vi "Bed_control.vi"(11 "pulse steps":i32=6436 min=4 step=1) -> ()   [LabVIEW 2019]
uses:
  <vilib>/DAQmx/write.llb/DAQmx Write (Digital 1D Wfm NChan NSamp).vi
  <vilib>/DAQmx/read.llb/DAQmx Read (Digital Bool 1Line 1Point).vi
  <vilib>/DAQmx/create/channels.llb/DAQmx Create Channel (DO-Digital Output).vi
  <vilib>/DAQmx/create/channels.llb/DAQmx Create Channel (DI-Digital Input).vi
  <vilib>/DAQmx/configure/timing.llb/DAQmx Timing (Sample Clock).vi
  <vilib>/Waveform/DWDTOps.llb/DWDT Digital Size.vi
  <vilib>/Waveform/DWDTOps.llb/DWDT Uncompress Digital.vi
  <vilib>/DAQmx/miscellaneous.llb/DAQmx Fill In Error Info.vi
  global_variables.vi
panel:
  out "travel distance (mm)":dbl=643.6
  in  "Move bed 2":bool
  in  "latch switch line":tag="DAQ1/port0/line3"
  out "Homing in progress":bool
  out "duration of movement":dbl=38.616
  in  "output lines":tag="DAQ1/port0/line0:2"
  in  "pulse duration (T/2)":dbl=0.003 format="%#_13p"
  out "Position":dbl(slide)=6836.0 scale=0.0..8000.0
  in  "Maximum absolute position":i32=8000 format="%.0p"
  out "Absolute position (pulses)":i32=6836
  in  "Abort movement":bool
  in  "Go home!":bool
  in  "Move bed":bool
  out "pulses to move":i32=6436
  in  "stop":bool
  # "DAQ settings"
  # "Homing"
  # "Enables PDU automatically"
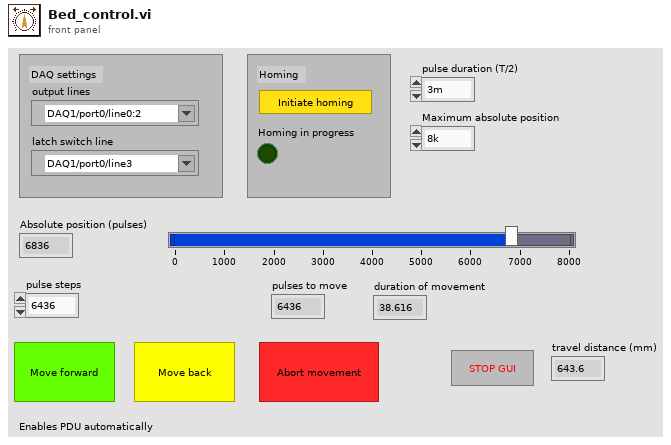
[diagram p1: front panel]
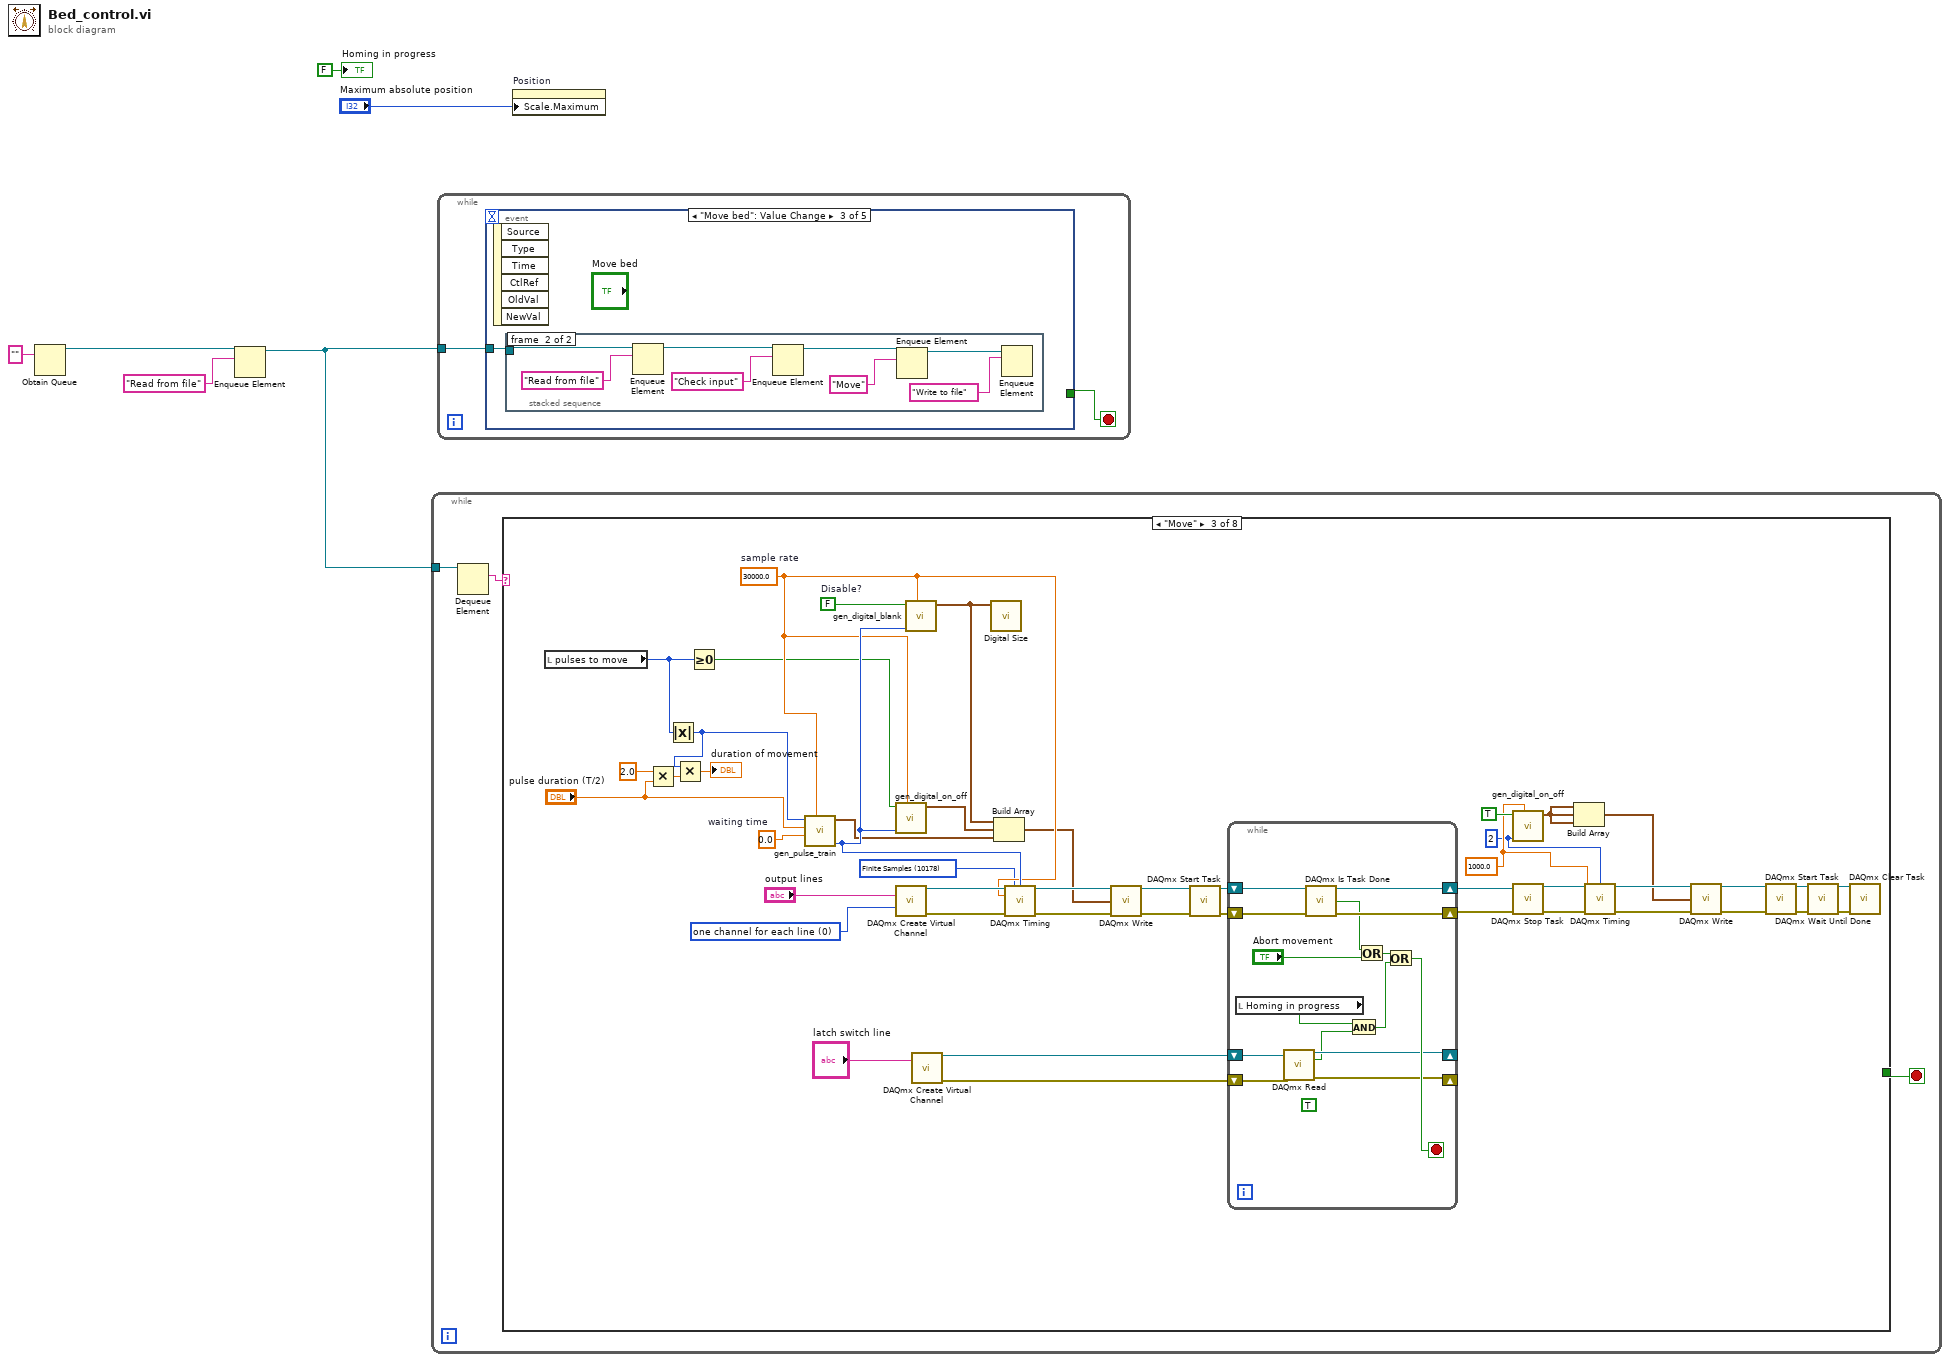
[diagram p0: block diagram]
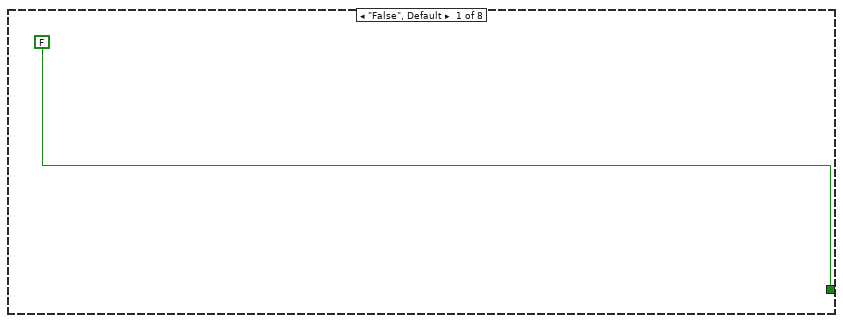
[diagram p2: hidden frame]
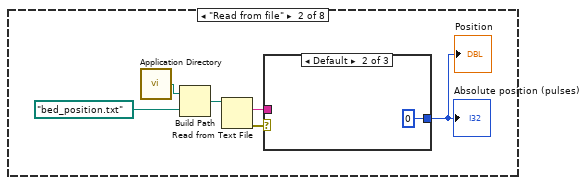
[diagram p3: hidden frame]
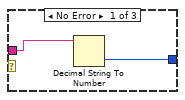
[diagram p4: hidden frame]
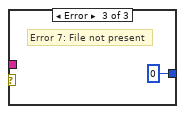
[diagram p5: hidden frame]
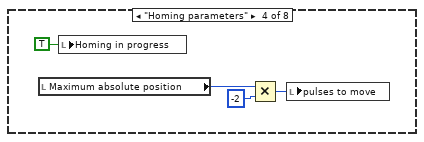
[diagram p6: hidden frame]
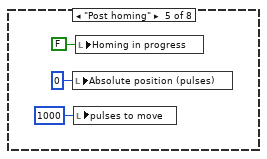
[diagram p7: hidden frame]
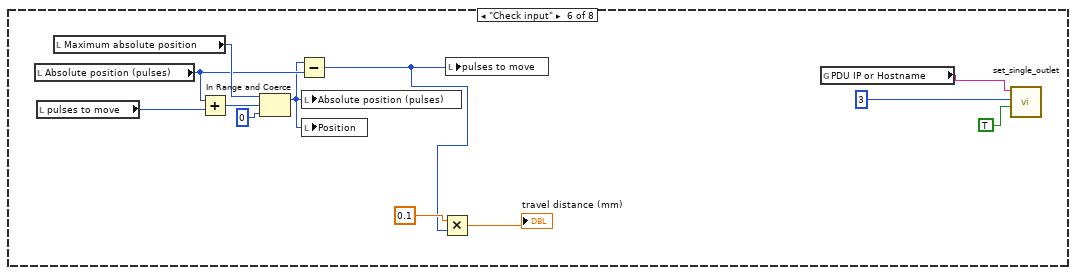
[diagram p8: hidden frame]
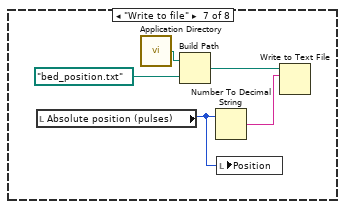
[diagram p9: hidden frame]
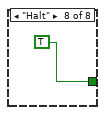
[diagram p10: hidden frame]
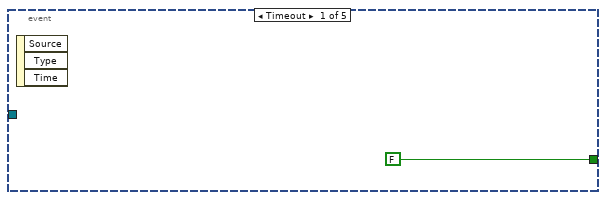
[diagram p11: hidden frame]
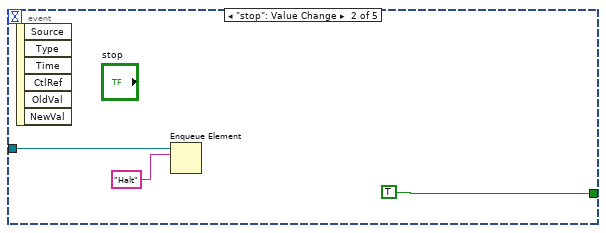
[diagram p12: hidden frame]
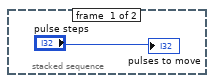
[diagram p13: hidden frame]
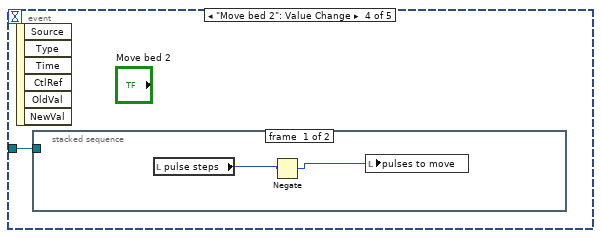
[diagram p14: hidden frame]
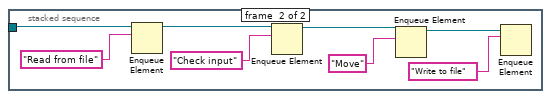
[diagram p15: hidden frame]
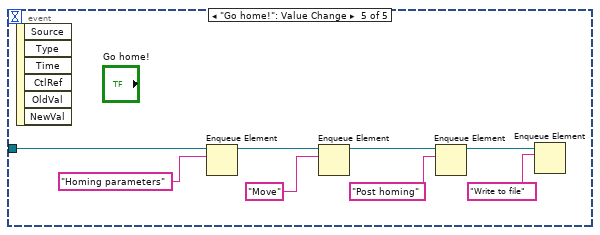
[diagram p16: hidden frame]
diagram:
  n1 = Obtain Queue(element data type="") -> (queue out=w5:refnum<queue>)  [unwired: 4 in, 2 out]
  n2 = Enqueue Element(queue=w5, element="Read from file") -> (queue out=w4:refnum<queue>)  [unwired: 2 in, 2 out]
  n3 = while {
    tunnel: w4 -> [w9]
    stop <- w7 stop-if-true
    n4 = Dequeue Element(queue=w9) -> (element=w8:string)  [unwired: 2 in, 3 out]
    n5 = case shown="\"Move\"" w8 {
      tunnel: [FALSE _ _ _ _ _ _ TRUE] -> w7
      frame "False", Default {
      }
      frame "Read from file" {
        n6 = call <vilib>:"Application Directory.vi"() -> ("Application Directory"=w13:path)
        n7 = Build Path(base path=w13, name or relative path=path "bed_position.txt" ("file (use dialog)")) -> (appended path=w14:path)
        n8 = Read from Text File(file (use dialog)=w14) -> (text=w16:string, error out=w15:errorcluster)  [unwired: 3 in, 2 out]
        n9 = case shown="Default" w15 {
          tunnel: w16 -> [w18 _ _]
          tunnel: [w17 0 0] -> w11
          frame No Error {
            n10 = Decimal String To Number(string=w18) -> (number=w17:i32)  [unwired: 2 in, 1 out]
          }
          frame Default {
          }
          frame Error {
            # "Error 7: File not present"
          }
        }
        "Absolute position (pulses)" <- w11
        "Position" <- w11
      }
      frame "Move" {
        w26 = 2 ("waveform length")
        w27 = 1000.0 ("rate")
        w51 = 0.0  # waiting time
        w56 = 30000.0  # sample rate
        w55 = FALSE  # Disable?
        w54 = 10178 items=["Finite Samples"=10178, "Continuous Samples"=10123, "Hardware Timed Single Point"=12522] ("sample mode")
        w52 = 0 items=["one channel for each line", "one channel for all lines"] ("line grouping")
        n11 = local read "pulses to move"() -> (w25:i32)
        n12 = Multiply(x=2.0, y="pulse duration (T/2)") -> (x*y=w47:dbl)
        n13 = Absolute Value(x=w25) -> (abs(x)=w48:i32)
        n14 = Multiply(x=w48, y=w47) -> (x*y=→"duration of movement":dbl)
        n15 = Greater Or Equal To 0?(x=w25) -> (x >= 0?=w50:bool)
        n16 = call "gen_pulse_train.vi"("sampling rate"=w56, "waiting time"=w51, "pulse width"="pulse duration (T/2)", "Number of pulses"=w48) -> ("waveform length"=w63:i32, "digital waveform out"=w61:digitalwaveform)  [unwired: 6 in]
        n17 = call "gen_digital_on_off.vi"("sampling rate"=w56, "waveform length"=w63, "On / Off"=w50) -> ("digital waveform"=w62:digitalwaveform)  [unwired: 8 in]
        n18 = call-poly <vilib>:"DAQmx Create Virtual Channel.vi"("lines"="output lines", "line grouping"=w52) -> ("task out"=w57:refnum<k21>, "error out"=w60:errorcluster)  [unwired: 12 in]
        n19 = call "gen_digital_blank.vi"("sampling rate"=w56, "waveform length"=w63, "On / Off"=w55) -> ("digital waveform"=w66:digitalwaveform)  [unwired: 8 in]
        n20 = call-poly <vilib>:"DAQmx Create Virtual Channel.vi"("lines"="latch switch line") -> ("task out"=w22:refnum<k21>, "error out"=w23:errorcluster)  [unwired: 13 in]
        n21 = call-poly <vilib>:"Digital Size.vi"("digital waveform in"=w66) -> ()  [unwired: 7 in, 4 out]
        n22 = Build Array(w66, w62, w61) -> (w21:digitalwaveform[])
        n23 = call-poly <vilib>:"DAQmx Timing.vi"("task/channels in"=w57, "sample mode"=w54, "samples per channel"=w63, "rate"=w56, "error in"=w60) -> ("task out"=w58:refnum<k21>, "error out"=w59:errorcluster)  [unwired: 9 in]
        n24 = call-poly <vilib>:"DAQmx Write.vi"("task/channels in"=w58, "data"=w21, "error in"=w59) -> ("task out"=w64:refnum<k21>, "error out"=w65:errorcluster)  [unwired: 10 in, 1 out]
        n25 = call <vilib>:"DAQmx Start Task.vi"("task/channels in"=w64, "error in"=w65) -> ("task out"=w44:refnum<k21>, "error out"=w43:errorcluster)  [unwired: 12 in]
        n26 = while {
          shift-right: [w78] -> w41
          shift-left: w43 -> [w80]
          shift-right: [w79] -> w42
          shift-left: w44 -> [w81]
          shift-right: [w70] -> _
          shift-left: w22 -> [w73]
          shift-right: [w71] -> _
          shift-left: w23 -> [w72]
          stop <- w74 stop-if-true
          (unwired) TRUE ("Abort movement")
          n27 = local read "Homing in progress"() -> (w69:bool)
          n28 = call-poly <vilib>:"DAQmx Read.vi"("task/channels in"=w73, "error in"=w72) -> ("task out"=w70:refnum<k21>, "data"=w67:bool, "error out"=w71:errorcluster)  [unwired: 11 in]
          n29 = call <vilib>:"DAQmx Is Task Done.vi"("task/channels in"=w81, "error in"=w80) -> ("task out"=w79:refnum<k21>, "task done?"=w76:bool, "error out"=w78:errorcluster)  [unwired: 11 in]
          n30 = And(x=w69, y=w67) -> (x .and. y?=w68:bool)
          n31 = Or(x=w76, y="Abort movement") -> (x .or. y?=w75:bool)
          n32 = Or(x=w75, y=w68) -> (x .or. y?=w74:bool)
        }
        n33 = call "gen_digital_on_off.vi"("sampling rate"=w27, "waveform length"=w26, "On / Off"=TRUE) -> ("digital waveform"=w30:digitalwaveform)  [unwired: 8 in]
        n34 = call <vilib>:"DAQmx Stop Task.vi"("task/channels in"=w42, "error in"=w41) -> ("task out"=w31:refnum<k21>, "error out"=w34:errorcluster)  [unwired: 12 in]
        n35 = Build Array(w30, w30, w30) -> (w29:digitalwaveform[])
        n36 = call-poly <vilib>:"DAQmx Timing.vi"("task/channels in"=w31, "samples per channel"=w26, "rate"=w27, "error in"=w34) -> ("task out"=w32:refnum<k21>, "error out"=w33:errorcluster)  [unwired: 10 in]
        n37 = call-poly <vilib>:"DAQmx Write.vi"("task/channels in"=w32, "data"=w29, "error in"=w33) -> ("task out"=w40:refnum<k21>, "error out"=w39:errorcluster)  [unwired: 10 in, 1 out]
        n38 = call <vilib>:"DAQmx Start Task.vi"("task/channels in"=w40, "error in"=w39) -> ("task out"=w38:refnum<k21>, "error out"=w37:errorcluster)  [unwired: 12 in]
        n39 = call <vilib>:"DAQmx Wait Until Done.vi"("task/channels in"=w38, "error in"=w37) -> ("task out"=w36:refnum<k21>, "error out"=w35:errorcluster)  [unwired: 12 in]
        n40 = call <vilib>:"DAQmx Clear Task.vi"("task in"=w36, "error in"=w35) -> ()  [unwired: 13 in, 1 out]
      }
      frame "Homing parameters" {
        n41 = local read "Maximum absolute position"() -> (w84:i32)
        n42 = local write "Homing in progress"(TRUE ("Homing in progress")) -> ()
        n43 = Multiply(x=w84, y=-2) -> (x*y=w82:i32)
        n44 = local write "pulses to move"(w82) -> ()
      }
      frame "Post homing" {
        n45 = local write "Absolute position (pulses)"(0 ("Absolute position (pulses)")) -> ()
        n46 = local write "pulses to move"(1000 ("pulses to move")) -> ()
        n47 = local write "Homing in progress"(FALSE ("Homing in progress")) -> ()
      }
      frame "Check input" {
        n48 = local read "Absolute position (pulses)"() -> (w98:i32)
        n49 = local read "pulses to move"() -> (w95:i32)
        n50 = local read "Maximum absolute position"() -> (w99:i32)
        n51 = Add(x=w98, y=w95) -> (x+y=w100:i32)
        n52 = In Range and Coerce(upper limit=w99, x=w100, lower limit=0) -> (coerced(x)=w97:i32)  [unwired: 1 out]
        n53 = Subtract(x=w97, y=w98) -> (x-y=w92:i32)
        n54 = local write "Absolute position (pulses)"(w97) -> ()
        n55 = local write "Position"(w97) -> ()
        n56 = Multiply(x=0.1, y=w92) -> (x*y=→"travel distance (mm)":dbl)
        n57 = local write "pulses to move"(w92) -> ()
        n58 = global read "global_variables.vi" "PDU IP or Hostname"() -> (w91:string)
        n59 = call "set_single_outlet.vi"("Switch state"=TRUE, "Outlet #"=3, "IP / Hostname"=w91) -> ()  [unwired: 9 in]
      }
      frame "Write to file" {
        n60 = local read "Absolute position (pulses)"() -> (w101:i32)
        n61 = call <vilib>:"Application Directory.vi"() -> ("Application Directory"=w105:path)
        n62 = Build Path(base path=w105, name or relative path=path "bed_position.txt" ("file (use dialog)")) -> (appended path=w104:path)
        n63 = Number To Decimal String(number=w101) -> (decimal integer string=w103:string)  [unwired: 1 in]
        n64 = local write "Position"(w101) -> ()
        n65 = Write to Text File(file (use dialog)=w104, text=w103) -> ()  [unwired: 2 in, 3 out]
      }
      frame "Halt" {
      }
    }
  }
  n66 = while {
    tunnel: w4 -> [w108]
    stop <- w107 stop-if-true
    n67 = event shown="[2] \"Move bed\": Value Change" {
      selector: _ -> [_ _ _ _ _]
      dyn-events: _ -> [_ _ _ _ _]
      timeout: _ -> [_ _ _ _ _]
      tunnel: w108 -> [_ w112 w113 w123 w140]
      tunnel: [FALSE TRUE _ _ _] -> w107
      event Timeout {
        n68 = event-data() -> ()  [unwired: 1 in, 3 out]
      }
      event "stop": Value Change {
        n69 = event-data() -> ()  [unwired: 1 in, 6 out]
        n70 = Enqueue Element(queue=w112, element="Halt") -> ()  [unwired: 2 in, 3 out]
      }
      event "Move bed": Value Change {
        n71 = event-data() -> ()  [unwired: 1 in, 6 out]
        n72 = stacked-sequence {
          tunnel: w113 -> [_ w122]
          frame #0 {
            "pulses to move" <- "pulse steps"
          }
          frame #1 {
            n73 = Enqueue Element(queue=w122, element="Read from file") -> (queue out=w116:refnum<queue>)  [unwired: 2 in, 2 out]
            n74 = Enqueue Element(queue=w116, element="Check input") -> (queue out=w115:refnum<queue>)  [unwired: 2 in, 2 out]
            n75 = Enqueue Element(queue=w115, element="Move") -> (queue out=w119:refnum<queue>)  [unwired: 2 in, 2 out]
            n76 = Enqueue Element(queue=w119, element="Write to file") -> ()  [unwired: 2 in, 3 out]
          }
        }
      }
      event "Move bed 2": Value Change {
        n77 = event-data() -> ()  [unwired: 1 in, 6 out]
        n78 = stacked-sequence {
          tunnel: w123 -> [_ w133]
          frame #0 {
            n79 = local read "pulse steps"() -> (w125:i32)
            n80 = Negate(x=w125) -> (-x=w124:i32)
            n81 = local write "pulses to move"(w124) -> ()
          }
          frame #1 {
            n82 = Enqueue Element(queue=w133, element="Read from file") -> (queue out=w127:refnum<queue>)  [unwired: 2 in, 2 out]
            n83 = Enqueue Element(queue=w127, element="Check input") -> (queue out=w126:refnum<queue>)  [unwired: 2 in, 2 out]
            n84 = Enqueue Element(queue=w126, element="Move") -> (queue out=w130:refnum<queue>)  [unwired: 2 in, 2 out]
            n85 = Enqueue Element(queue=w130, element="Write to file") -> ()  [unwired: 2 in, 3 out]
          }
        }
      }
      event "Go home!": Value Change {
        n86 = event-data() -> ()  [unwired: 1 in, 6 out]
        n87 = Enqueue Element(queue=w140, element="Homing parameters") -> (queue out=w137:refnum<queue>)  [unwired: 2 in, 2 out]
        n88 = Enqueue Element(queue=w137, element="Move") -> (queue out=w135:refnum<queue>)  [unwired: 2 in, 2 out]
        n89 = Enqueue Element(queue=w135, element="Post homing") -> (queue out=w134:refnum<queue>)  [unwired: 2 in, 2 out]
        n90 = Enqueue Element(queue=w134, element="Write to file") -> ()  [unwired: 2 in, 3 out]
      }
    }
  }
  n91 = property on="Position" class="Slide (strict)"("Scale.Maximum"="Maximum absolute position") -> ()  [unwired: 2 in, 2 out]
  "Homing in progress" <- FALSE ("Homing in progress")
